vi "initOCR.vi"(8 "error in (no error)":errorcluster, 10 "adsBase.lvlib:adsBase.lvclass":refnum<class "adsBase.lvclass">, 11 "ocr in":refnum<class "ocr.lvclass">) -> (0 "error out":errorcluster, 3 "ocr out":refnum<class "ocr.lvclass">)   [LabVIEW 2025, in "adsOCR.lvlib" / "ocr.lvclass"]
uses:
  ocr.lvclass
  ocr.lvclass/ocr.ctl
  adsBase/adsBase.lvclass
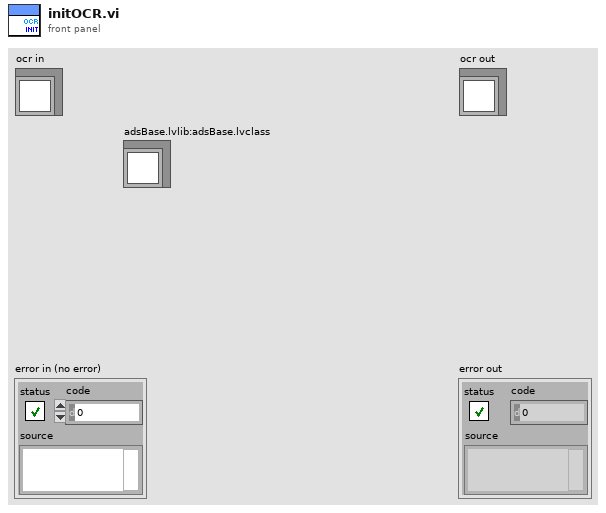
[diagram p1: front panel]
types:
  T1 = typedef "adsBase.lvlib/adsBase.lvclass/common.ctl" = cluster{"tcv":u64, "Path":path, "ResourcePath":string, "device":T2}
  T2 = typedef "adsBase.lvlib/adsBase.lvclass/devices.ctl" = enum16{"CPU", "GPU0"}
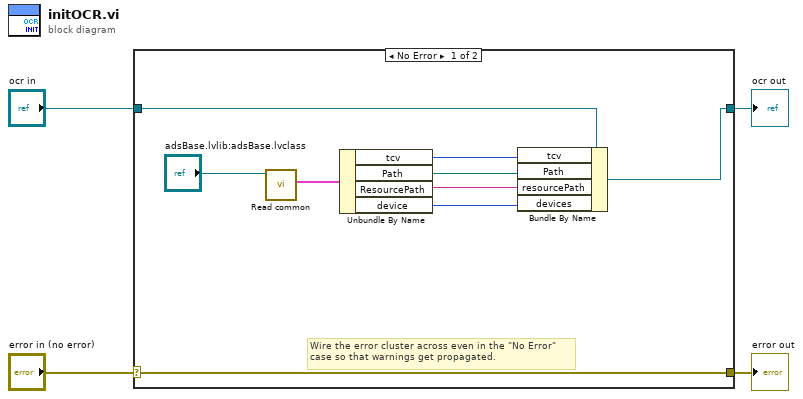
[diagram p0: block diagram]
diagram:
  n1 = case shown="No Error" "error in (no error)" {
    selector: "error in (no error)" -> [w13 w15]
    tunnel: [w13 w15] -> w3
    tunnel: [w5 w14] -> w1
    tunnel: "ocr in" -> [w10 w14]
    frame No Error {
      # "Wire the error cluster across even in the \"No Error\"\ncase so that warnings get propagated."
      n2 = call-dynamic "Read common.vi"("adsBase in"="adsBase.lvlib:adsBase.lvclass") -> ("common"=w11:T1)  [unwired: 8 in, 2 out]
      n3 = Unbundle By Name(w11) -> ("tcv"=w9:u64, "Path"=w8:path, "ResourcePath"=w7:string, "device"=w6:T2)
      n4 = Bundle By Name(cluster=w10, "tcv"=w9, "Path"=w8, "resourcePath"=w7, "devices"=w6) -> (w5:refnum<class "ocr.lvclass">)
    }
    frame Error {
    }
  }
  "error out" <- w3
  "ocr out" <- w1
